vi "DataWriteGen.vi"(0 "DataFileName":path, 5 "LastScanPosIn":dbl[](array[numeric]), 7 "XY Graph":T1(array[cluster]), 9 "AllYDataIn":dbl[][](array[numeric]), 11 "error in (no error)":errorcluster) -> (8 "XY Graph Out":T1(array[cluster]), 10 "AllYDataOut":dbl[][](array[numeric]), 15 "error out":errorcluster)   [LabVIEW 2010]
doc: "Ce VI sauvegarde les données d'acquisition pour en garder une copie de sécurité qui peut être rappeller en cas de panne."
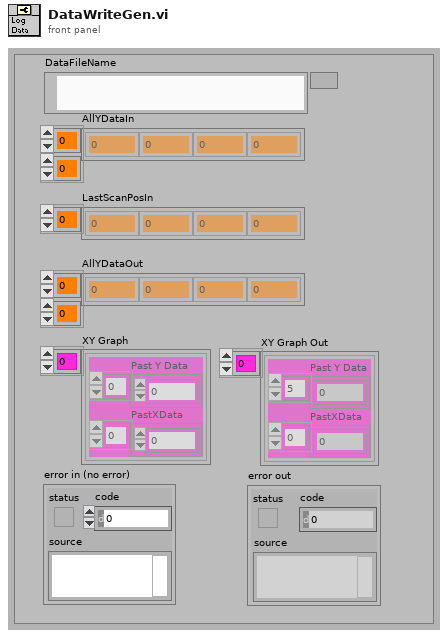
[diagram p1: front panel]
types:
  T1 = cluster{"Past Y Data":dbl[], "PastXData":dbl[]}[]
  T2 = cluster{"AllYDataIn":dbl[][], "XY Graph":cluster{"Past Y Data":dbl[], "PastXData":dbl[]}[], "LastScanPosIn":dbl[]}
  T3 = enum16{"open", "replace", "create", "open or create", "replace or create", "replace or create with confirmation"}
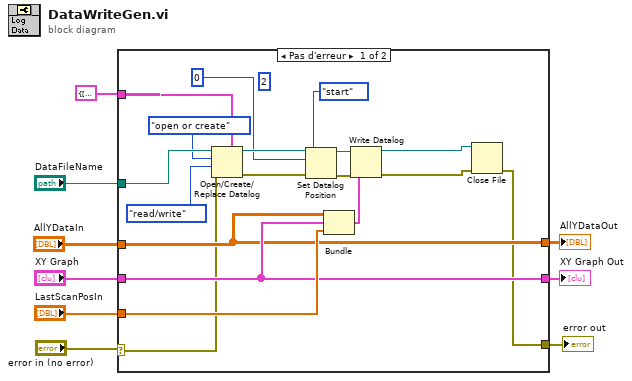
[diagram p0: block diagram]
diagram:
  n1 = case shown="Pas d'erreur" "error in (no error)" {
    selector: "error in (no error)" -> [w21 w30]
    tunnel: "LastScanPosIn" -> [w27 _]
    tunnel: "AllYDataIn" -> [w25 w29]
    tunnel: "XY Graph" -> [w26 w28]
    tunnel: [w18 w30] -> w5
    tunnel: [w26 w28] -> w4
    tunnel: [w25 w29] -> w3
    tunnel: "DataFileName" -> [w24 _]
    tunnel: T2 {"AllYDataIn"=[], "XY Graph"=[], "LastScanPosIn"=[]} -> [w22 _]
    frame No Error {
      (unwired) 2
      n2 = Open/Create/Replace Datalog(5:w22, 8:w21, 9:enum16{"read/write", "read-only", "write-only"}."read/write" ("accès (0 : read/write)"), 10:T3."open or create" ("opération (0 : open)"), 11:w24) -> (0:w15:errorcluster, 3:w14:refnum<k1>)  [unwired: 1 in, 1 out]
      n3 = Set Datalog Position(4:w15, 5:enum16{"start", "end", "current"}."start" ("à partir de (0 : start)"), 6:i64 0 ("offset (en nb d'enregistrements) (0)"), 7:w14) -> (0:w12:errorcluster, 3:w11:refnum<k1>)
      n4 = Bundle("AllYDataIn"=w25, "XY Graph"=w26, "LastScanPosIn"=w27) -> (w23:T2)  [unwired: 1 in]
      n5 = Write Datalog(4:w12, 6:w23, 7:w11) -> (0:w19:errorcluster, 3:w20:refnum<k1>)
      n6 = Close File(refnum=w20, error in=w19) -> (error out=w18:errorcluster)  [unwired: 1 out]
    }
    frame Error {
    }
  }
  "AllYDataOut" <- w3
  "XY Graph Out" <- w4
  "error out" <- w5
